vi "例程28-配置文件的读取.vi"() -> ()   [LabVIEW 2016]
uses:
  <vilib>/Utility/config.llb/Read Key (Boolean).vi
  <vilib>/Utility/config.llb/Read Key (String).vi
  <vilib>/Utility/config.llb/Read Key (Path).vi
  <vilib>/Utility/config.llb/Read Key (Double).vi
  <vilib>/Utility/config.llb/NI_LVConfig.lvlib
panel:
  out "字符串 2":string
  out "字符串":string
  out "路径":path
  out "数值":dbl
  out "布尔":bool
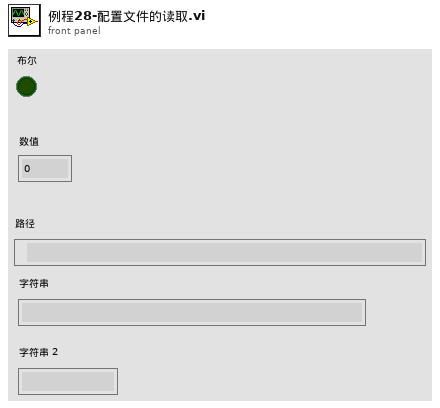
[diagram p1: front panel]
types:
  T1 = typedef "NI_LVConfig.lvlib/Config Data RefNum.ctl" = refnum<k1>
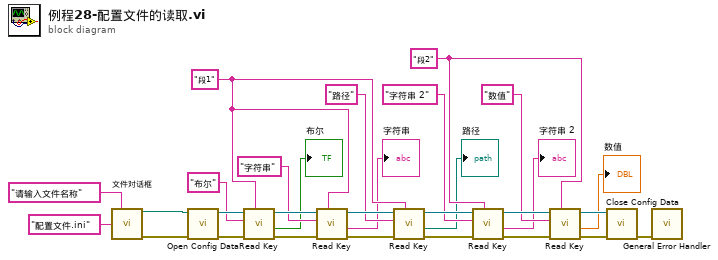
[diagram p0: block diagram]
diagram:
  w10 = "段2" ("section")
  w15 = "段1" ("section")
  n1 = call "文件对话框"("prompt"="请输入文件名称", "default name"="配置文件.ini") -> ("selected path"=w26:path, "error out"=w25:errorcluster)  [unwired: 10 in, 2 out]
  n2 = call <vilib>:"Open Config Data.vi"("error in (no error)"=w25, "configuration file path"=w26) -> ("error out"=w23:errorcluster, "refnum"=w24:T1)  [unwired: 7 in, 1 out]
  n3 = call-poly <vilib>:"Read Key.vi"("section"=w15, "error in (no error)"=w23, "key"="布尔", "refnum"=w24) -> ("error out"=w14:errorcluster, "value"=→"布尔":bool, "refnum out"=w13:T1)  [unwired: 4 in, 1 out]
  n4 = call-poly <vilib>:"Read Key.vi"("section"=w15, "error in (no error)"=w14, "key"="字符串", "refnum"=w13) -> ("error out"=w22:errorcluster, "value"=→"字符串":string, "refnum out"=w21:T1)  [unwired: 4 in, 1 out]
  n5 = call-poly <vilib>:"Read Key.vi"("section"=w15, "error in (no error)"=w22, "key"="路径", "refnum"=w21) -> ("error out"=w20:errorcluster, "value"=→"路径":path, "refnum out"=w19:T1)  [unwired: 4 in, 1 out]
  n6 = call-poly <vilib>:"Read Key.vi"("section"=w10, "error in (no error)"=w20, "key"="字符串 2", "refnum"=w19) -> ("error out"=w18:errorcluster, "value"=→"字符串 2":string, "refnum out"=w17:T1)  [unwired: 4 in, 1 out]
  n7 = call-poly <vilib>:"Read Key.vi"("section"=w10, "error in (no error)"=w18, "key"="数值", "refnum"=w17) -> ("error out"=w11:errorcluster, "value"=→"数值":dbl, "refnum out"=w9:T1)  [unwired: 4 in, 1 out]
  n8 = call <vilib>:"Close Config Data.vi"("error in (no error)"=w11, "refnum"=w9) -> ("error out"=w29:errorcluster)  [unwired: 8 in, 1 out]
  n9 = call <vilib>:"General Error Handler.vi"("error in (no error)"=w29) -> ()  [unwired: 10 in, 5 out]
